vi "intake sub Controller.vi"(8 "error in":errorcluster) -> ()   [LabVIEW 2020]
uses:
  <vilib>/Rock Robotics/WPI/Framework/Completion Status.ctl
  intake sub Setpoints.ctl
  intake sub Operations.ctl
  Typedef/intake typedef.ctl
  <vilib>/Rock Robotics/WPI/ThirdParty/REV Robotics/REVLib/Typedef/Spark MAX Control Type.ctl
  manipulator/Implementation/Typedefs/game object.ctl
  Framework/Robot Global Data.vi
  <vilib>/ptbypt/NI_PtbyPt.lvlib
  <vilib>/Rock Robotics/Network Tables/NT Write Boolean.vi
panel:
  out "Waveform Chart":dbl(graph)
  out "Current\nCmd":string
  in  "Buttons":cluster{"Execute Cmd":bool, "Abort Cmd":bool}
  out "Command Timing":cluster{"Start Time (ms)":u32, "Iterations":i32}
  out "Status":T1
  # "Interactive Command: You may fill in the settings for a command\nand schedule it with the Execute button. You can observe and abort\nany command while fine tuning the code for the controller."
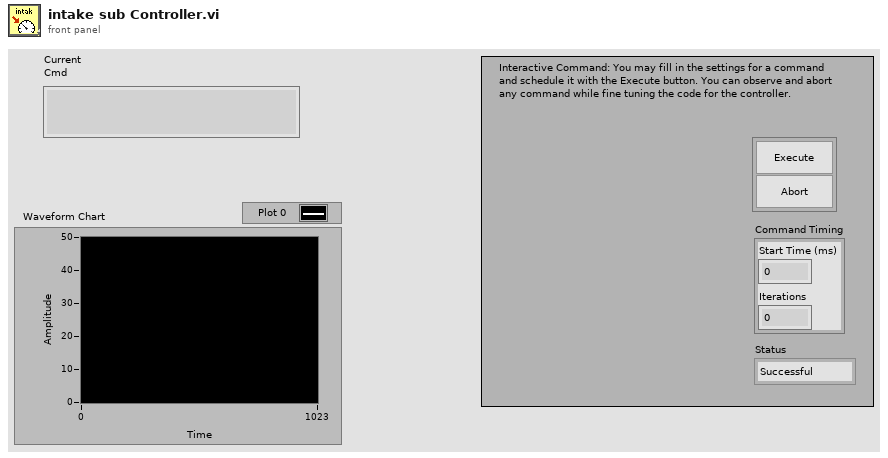
[diagram p1: front panel]
types:
  T1 = typedef "Completion Status.ctl" = enum16{"Successful", "Aborted", "Incomplete"}
  T2 = typedef "intake sub Setpoints.ctl" = cluster{"Operation":T3, "intake modes":T4}
  T3 = typedef "intake sub Operations.ctl" = enum16{"Reserve", "Read Current", "Immediate"}
  T4 = typedef "intake typedef.ctl" = enum16{"Intake Cone Sideways", "Intake Cone Upright", "Intake Cube", "Outtake/Score", "Shoot"}
  T5 = typedef "WPI_MotorControlDeviceRef.ctl" = cluster{"DeviceStatus":errorcluster, "Type":T6, "PWM":cluster{"PWM Channel":T7, "DeadBand":T8}, "CAN":cluster{"Device Number":u8, "SetOutput VI Ref":variant, "GetOutput VI Ref":variant, "Enable VI Ref":variant, "Disable VI Ref":variant, "Data":variant}, "Invert":bool, "DIO PWM":cluster{"PWM \"Enable\" Channel":T7, "DIOChannel":T9, "PWM Rate":dbl}}
  T6 = typedef "WPI_MotorControlType.ctl" = enum16{"PWM", "CAN", "DIO PWM"}
  T7 = typedef "FPGA_DIOPWMChannel.ctl" = enum8{"PWM 0", "PWM 1", "PWM 2", "PWM 3", "PWM 4", "PWM 5", "PWM 6", "PWM 7", "PWM 8", "PWM 9", "PWM MXP 0", "PWM MXP 1", "PWM MXP 2", "PWM MXP 3", "PWM MXP 4", "PWM MXP 5", "PWM MXP 6", "PWM MXP 7", "PWM MXP 8", "PWM MXP 9", "Invalid"}
  T8 = typedef "WPI_PWMDeadband.ctl" = cluster{"Name":string, "maxPositivePwm":i32, "minPositivePwm":i32, "centerPwm":i32, "maxNegativePwm":i32, "minNegativePwm":i32, "angularRange":u16}
  T9 = typedef "FPGA_DIOChannel.ctl" = enum8{"DIO 0", "DIO 1", "DIO 2", "DIO 3", "DIO 4", "DIO 5", "DIO 6", "DIO 7", "DIO 8", "DIO 9", "DIO MXP 0", "DIO MXP 1", "DIO MXP 2", "DIO MXP 3", "DIO MXP 4", "DIO MXP 5", "DIO MXP 6", "DIO MXP 7", "DIO MXP 8", "DIO MXP 9", "DIO MXP 10", "DIO MXP 11", "DIO MXP 12", "DIO MXP 13", "DIO MXP 14", "DIO MXP 15", "SPI Port CS1", "SPI Port CS2", "SPI Port CS3", "SPI Port MISO", "SPI Port MOSI", "Invalid"}
  T10 = typedef "Command Status Info.ctl" = cluster{"Name":string, "Status":T1, "notifier out":T11}
  T11 = typedef "Completion Notifier.ctl" = refnum<notifier>
  T12 = cluster{"Current Command":T2, "Command Timing":cluster{"Start Time (ms)":u32, "Iterations":i32}, "Command Arguments":cluster{"Command Info":T10, "Description":string, "Default Command":T2, "queue out":refnum<queue>, "Subsystem Name":string}}
  T13 = typedef "Spark MAX Control Type.ctl" = enum16{"Percent VBus", "Voltage", "Velocity", "Position", "Smart Motion", "Current", "Smart Velocity"}
  T14 = typedef "game object.ctl" = enum16{"Nothing", "Cone", "Cube"}
  T15 = cluster{"Preset Name":string, "Cone":dbl, "Cube":dbl}[]
  T16 = cluster{"Preset Name":string, "Cone":dbl, "Cube":dbl}
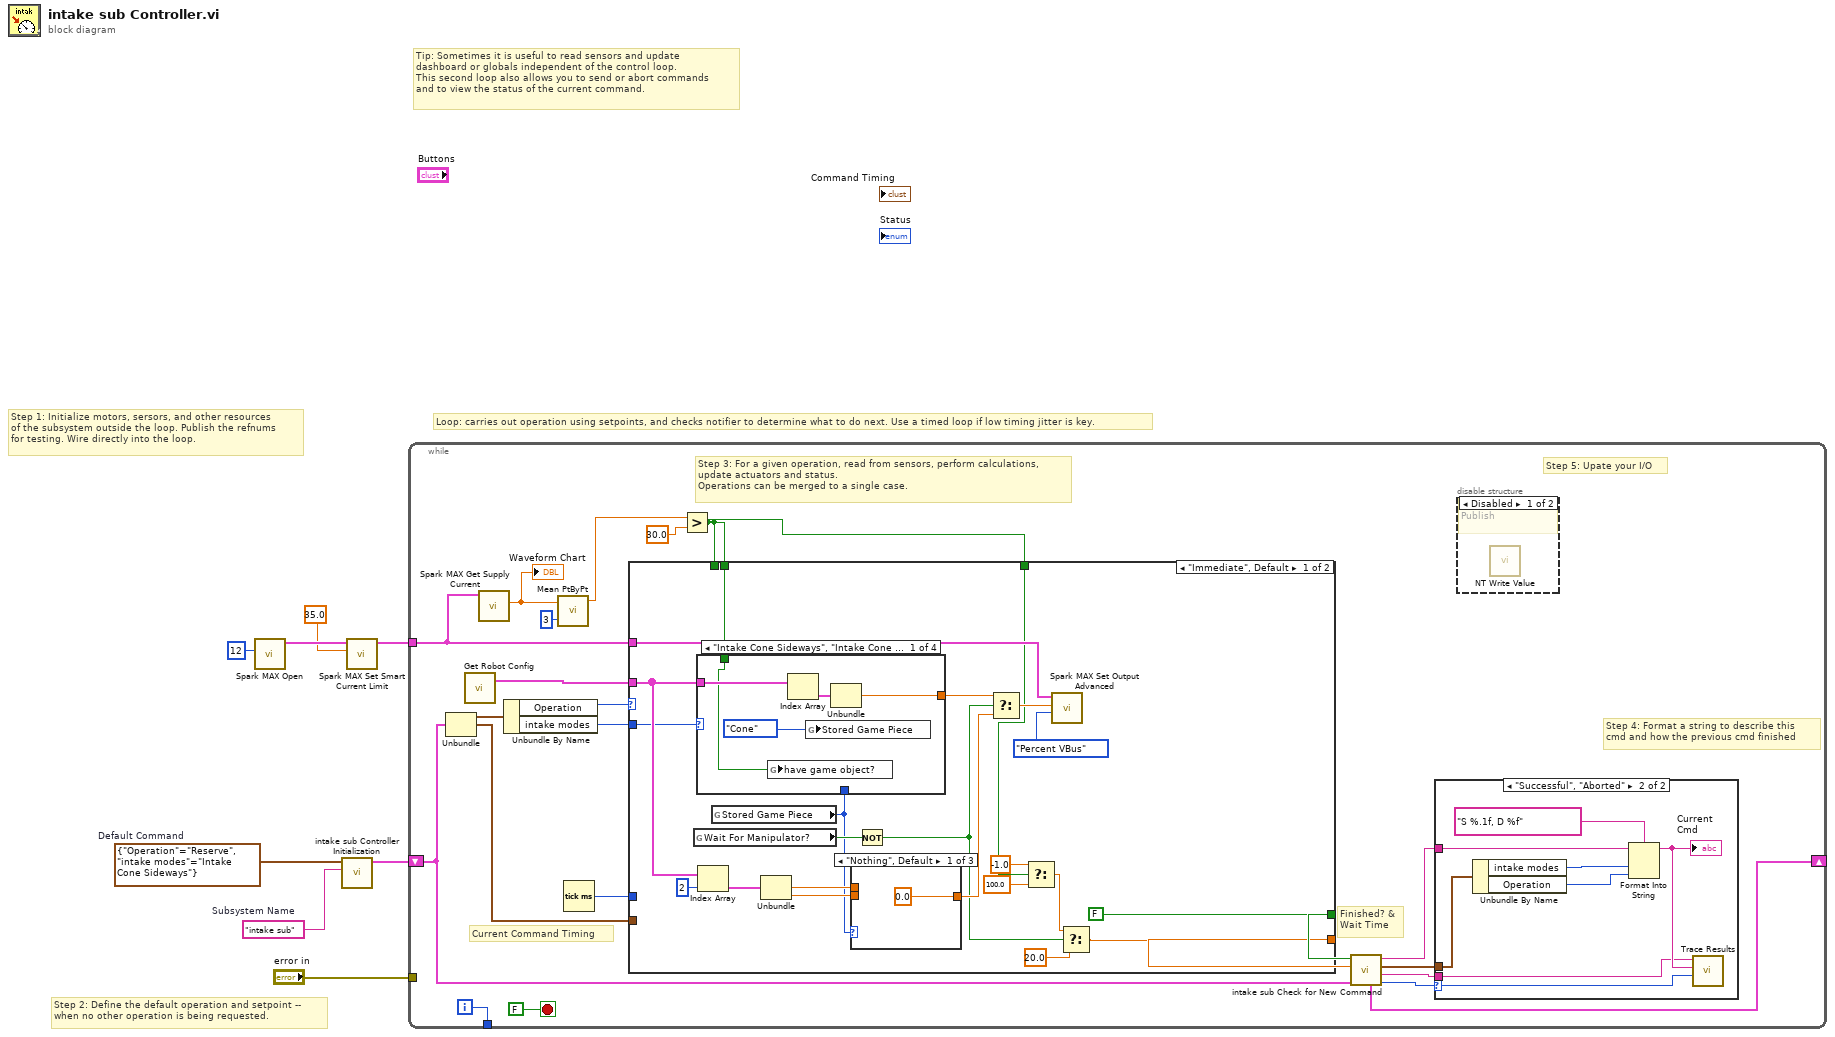
[diagram p0: block diagram]
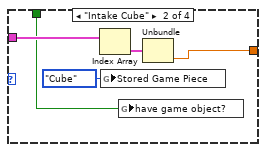
[diagram p6: hidden frame]
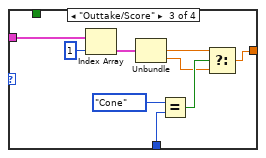
[diagram p7: hidden frame]
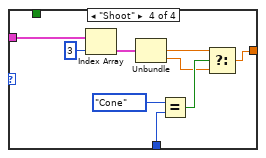
[diagram p8: hidden frame]
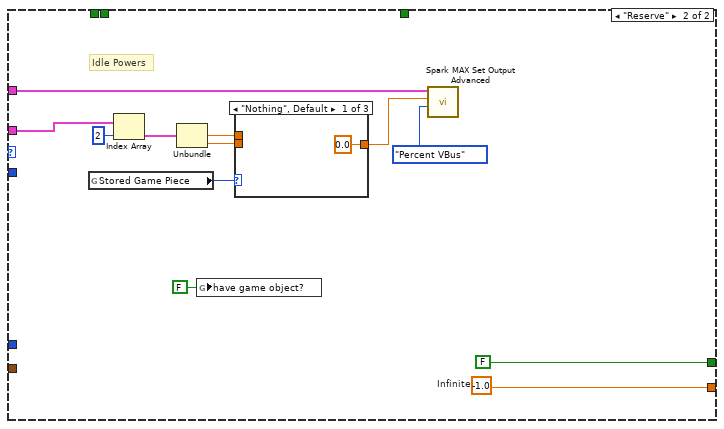
[diagram p9: hidden frame]
diagram:
  w5 = T2 {"Operation"=enum."Reserve", "intake modes"=enum."Intake Cone Sideways"}  # Default Command
  w6 = "intake sub"  # Subsystem Name
  # "Tip: Sometimes it is useful to read sensors and update\ndashboard or globals independent of the control loop.\nThis second loop also allows you to send or abort commands\nand to view the status of the current command."
  # "Step 2: Define the default operation and setpoint --\nwhen no other operation is being requested."
  # "Step 1: Initialize motors, sersors, and other resources\nof the subsystem outside the loop. Publish the refnums\nfor testing. Wire directly into the loop."
  # "Loop: carries out operation using setpoints, and checks notifier to determine what to do next. Use a timed loop if low timing jitter is key."
  n1 = call <vilib>:"Spark MAX Open.vi"("Device Number"=u8 12) -> ("MotorControlDeviceRef"=w3:T5)  [unwired: 9 in, 1 out]
  n2 = call "intake sub Controller Initialization.vi"("Subsystem Name"=w6, "Default Command"=w5) -> ("Current Command"=w7:T12)  [unwired: 9 in]
  n3 = call <vilib>:"Spark MAX Set Smart Current Limit.vi"("Primay Current Limit (80A)"=35.0, "MotorControlDeviceRef in"=w3) -> ("MotorControlDeviceRef out"=w2:T5)  [unwired: 8 in, 1 out]
  n4 = while {
    shift-right: [w23] -> _
    shift-left: w7 -> [w16]
    tunnel: [w29] -> _
    tunnel: "error in" -> [_]
    tunnel: w2 -> [w15]
    i -> [w29]
    stop <- FALSE stop-if-true
    # "Step 5: Upate your I/O"
    # "Step 4: Format a string to describe this\ncmd and how the previous cmd finished"
    # "Current Command Timing"
    # "Finished? &\nWait Time"
    # "Step 3: For a given operation, read from sensors, perform calculations,\nupdate actuators and status.\nOperations can be merged to a single case."
    n5 = Unbundle(w16) -> ("Current Command"=w28:T2, "Command Timing"=w24:cluster{"Start Time (ms)":u32, "Iterations":i32})  [unwired: 1 out]
    n6 = call "Get Robot Config.vi"() -> ("Intake Presets"=w14:T15)  [unwired: 12 in, 7 out]
    n7 = call <vilib>:"Spark MAX Get Supply Current.vi"("MotorControlDevRef in"=w15) -> ("Current"=w12:dbl)  [unwired: 7 in, 3 out]
    "Waveform Chart" <- w12
    n8 = Unbundle By Name(w28) -> ("Operation"=w27:T3, "intake modes"=w26:T4)
    n9 = call <vilib>:"Mean PtByPt.vi"("x"=w12, "sample length"=3) -> ("mean"=w11:dbl)  [unwired: 2 in, 1 out]
    n10 = Tick Count (ms)() -> (millisecond timer value=w25:u32)
    n11 = Greater?(x=w11, y=30.0 ("current")) -> (0:w9:bool)
    n12 = case shown="\"Immediate\", Default" w27 {
      tunnel: [w47 w103] -> w21
      tunnel: [FALSE ("ignore previous (F)") FALSE ("ignore previous (F)")] -> w22
      tunnel: w24 -> [_ _]
      tunnel: w26 -> [w40 _]
      tunnel: w25 -> [_ _]
      tunnel: w15 -> [w56 w93]
      tunnel: w14 -> [w50 w101]
      tunnel: w9 -> [w43 _]
      tunnel: w9 -> [_ _]
      tunnel: w9 -> [w39 _]
      frame "Immediate", Default {
        n13 = global read "Robot Global Data.vi" "Wait For Manipulator?"() -> (w55:bool)
        n14 = Index Array(array=w50, index=2) -> (element=w54:T16)
        n15 = global read "Robot Global Data.vi" "Stored Game Piece"() -> (w49:T14)
        n16 = case shown="\"Intake Cone Sideways\", \"Intake Cone Upright\"" w40 {
          tunnel: w50 -> [w68 w73 w82 w91]
          tunnel: [w66 w71 w75 w84] -> w58
          tunnel: w49 -> [_ _ w74 w83]
          tunnel: w39 -> [w64 w69 _ _]
          frame "Intake Cone Sideways", "Intake Cone Upright" {
            n17 = global write "Robot Global Data.vi" "have game object?"(w64) -> ()
            n18 = Index Array(array=w68) -> (element=w67:T16)  [unwired: 1 in]
            n19 = global write "Robot Global Data.vi" "Stored Game Piece"(game_object."Cone" ("Stored Game Piece")) -> ()
            n20 = Unbundle(w67) -> ("Cone"=w66:dbl)  [unwired: 2 out]
          }
          frame "Intake Cube" {
            n21 = Index Array(array=w73) -> (element=w72:T16)  [unwired: 1 in]
            n22 = global write "Robot Global Data.vi" "Stored Game Piece"(game_object."Cube" ("Stored Game Piece")) -> ()
            n23 = global write "Robot Global Data.vi" "have game object?"(w69) -> ()
            n24 = Unbundle(w72) -> ("Cube"=w71:dbl)  [unwired: 2 out]
          }
          frame "Outtake/Score" {
            n25 = Index Array(array=w82, index=1) -> (element=w80:T16)
            n26 = Unbundle(w80) -> ("Cone"=w79:dbl, "Cube"=w76:dbl)  [unwired: 1 out]
            n27 = Equal?(x=game_object."Cone" ("y"), y=w74) -> (x = y?=w77:bool)
            n28 = Select(t=w79, s=w77, f=w76) -> (s? t:f=w75:dbl)
          }
          frame "Shoot" {
            n29 = Index Array(array=w91, index=3) -> (element=w89:T16)
            n30 = Unbundle(w89) -> ("Cone"=w88:dbl, "Cube"=w85:dbl)  [unwired: 1 out]
            n31 = Equal?(x=game_object."Cone" ("y"), y=w83) -> (x = y?=w86:bool)
            n32 = Select(t=w88, s=w86, f=w85) -> (s? t:f=w84:dbl)
          }
        }
        n33 = Unbundle(w54) -> ("Cone"=w52:dbl, "Cube"=w51:dbl)  [unwired: 1 out]
        n34 = case shown="\"Nothing\", Default" w49 {
          tunnel: w52 -> [_ w62 _]
          tunnel: w51 -> [_ _ w63]
          tunnel: [0.0 ("Cube") w62 w63] -> w48
          frame "Nothing", Default {
          }
          frame "Cone" {
          }
          frame "Cube" {
          }
        }
        n35 = Not(x=w55) -> (.not. x?=w46:bool)
        n36 = Select(t=w58, s=w46, f=w48) -> (s? t:f=w57:dbl)
        n37 = Select(t=-1.0, s=w43, f=100.0) -> (s? t:f=w44:dbl)
        n38 = call <vilib>:"Spark MAX Set Output Advanced.vi"("Control Mode"=Spark_MAX_Control_Type."Percent VBus", "Setpoint"=w57, "MotorControlDevRef"=w56) -> ()  [unwired: 7 in, 2 out]
        n39 = Select(t=w44, s=w46, f=20.0) -> (s? t:f=w47:dbl)
      }
      frame "Reserve" {
        w103 = -1.0  # Infinite
        # "Idle Powers"
        n40 = global read "Robot Global Data.vi" "Stored Game Piece"() -> (w97:T14)
        n41 = Index Array(array=w101, index=2) -> (element=w100:T16)
        n42 = Unbundle(w100) -> ("Cone"=w96:dbl, "Cube"=w95:dbl)  [unwired: 1 out]
        n43 = global write "Robot Global Data.vi" "have game object?"(FALSE ("have game object?")) -> ()
        n44 = case shown="\"Nothing\", Default" w97 {
          tunnel: w96 -> [_ w105 _]
          tunnel: w95 -> [_ _ w106]
          tunnel: [0.0 ("Cube") w105 w106] -> w94
          frame "Nothing", Default {
          }
          frame "Cone" {
          }
          frame "Cube" {
          }
        }
        n45 = call <vilib>:"Spark MAX Set Output Advanced.vi"("Control Mode"=Spark_MAX_Control_Type."Percent VBus", "Setpoint"=w94, "MotorControlDevRef"=w93) -> ()  [unwired: 7 in, 2 out]
      }
    }
    n46 = call "intake sub Check for New Command.vi"("Current Command"=w16, "Wait time (ms)"=w21, "Finished?"=w22) -> ("Completion"=w17:T1, "Subsystem Name"=w18:string, "Current Command"=w19:T2, "Initial Trace String"=w20:string, "NextCommand"=w23:T12)  [unwired: 4 in]
    n47 = case shown="\"Successful\", \"Aborted\"" w17 {
      selector: w17 -> [_ w38]
      tunnel: w20 -> [_ w34]
      tunnel: w19 -> [_ w35]
      tunnel: w18 -> [_ w31]
      frame "Incomplete", Default {
        # "Continuing current command"
      }
      frame "Successful", "Aborted" {
        # "Report and setup for next command"
        n48 = Unbundle By Name(w35) -> ("intake modes"=w37:T4, "Operation"=w32:T3)
        n49 = Format Into String(format string="S %.1f, D %f", initial string=w34, w37, w32) -> (resulting string=w33:string)  [unwired: 1 in, 1 out]
        "Current\nCmd" <- w33
        n50 = call <vilib>:"Trace Results.vi"("Status of previous command"=w38, "Description"=w33, "Subsystem"=w31) -> ()  [unwired: 9 in]
      }
    }
    n51 = disable-structure shown="Disabled" {
      frame Disabled {
        # "Publish"
        n52 = call-poly <vilib>:"NT Write Value.vi"() -> ()  [unwired: 11 in, 1 out]
      }
      frame Enabled {
      }
    }
  }
